vi "dfd_Set MRate Model.vi"(4 "output rounding mode":T5 caption="output round-off mode", 5 "output integer word length":T1, 6 "internal precision":T7, 8 "input iwl":i16=1, 9 "output wl":i16=16, 10 "input wl":i16=16, 11 "multirate filter in":T2={"mMRate_Structure"=enum."CIC", "mMRate_Mode"=0, "mMRate_Factor"=1, "mMRate_FIRParams"={"mMRate_FIR_H"=[], "mMRate_FIR_IsNyquist?"=FALSE, "mMRate_FIR_IsSymmetric?"=FALSE}, "mMRate_CICParams"={"mMRate_CIC_#Stage"=2, "mMRate_CIC_Lag"=1, "mMRate_CIC_Type"=enum."Lowpass"}, "mMRate_Order"=0, "mMRate_Version"="1.0", "mMRate_Comments"="", "mMRate_RationalFactor"={"mMRate_L"=-1, "mMRate_M"=-1}, "mMRate_Fs"=1.0, "mMRate_Quantized?"=FALSE, "mMRate_QFilterGain"=1.0, "mMRate_CoefWl"=16, "mMRate_Scaling"={"mMRate_ScaleByPowerOf2?"=FALSE, "mMRate_ScaleType"=enum."Time Domain 1-Norm"}, "mMRate_InputWl"=0, "mMRate_OutputWl"=0, "mMRate_OutputMode"=enum."Nearest", "mMRate_MultMode"=enum."Truncated", "mMRate_BitPruning"=FALSE, "mMRate_GainWl"=16, "mMRate_OutputFwl"=0, "mMRate_SumIwl"=0, "mMRate_InputIwl "=16, "mMRate_SumWl"=32, "mMRate_CoefIwl"=0} {"mMRate_SumWl" min=1 max=32 step=1; "mMRate_InputIwl" min=1 max=32 step=1; "mMRate_GainWl" min=1 max=32 step=1; "mMRate_OutputWl" min=1 max=32 step=1; "mMRate_InputWl" min=1 max=32 step=1; "mMRate_CoefWl" min=1 max=32 step=1; "mMRate_Mode" items=["Default"=-1, "No Rate Change"=0, "Interpolation"=1, "Decimation"=2, "Interpolated"=3, "Rational"=4]}) -> (3 "multirate filter out":T2={"mMRate_Structure"=enum."CIC", "mMRate_Mode"=0, "mMRate_Factor"=1, "mMRate_FIRParams"={"mMRate_FIR_H"=[], "mMRate_FIR_IsNyquist?"=FALSE, "mMRate_FIR_IsSymmetric?"=FALSE}, "mMRate_CICParams"={"mMRate_CIC_#Stage"=2, "mMRate_CIC_Lag"=1, "mMRate_CIC_Type"=enum."Lowpass"}, "mMRate_Order"=0, "mMRate_Version"="1.0", "mMRate_Comments"="", "mMRate_RationalFactor"={"mMRate_L"=-1, "mMRate_M"=-1}, "mMRate_Fs"=1.0, "mMRate_Quantized?"=FALSE, "mMRate_QFilterGain"=1.0, "mMRate_CoefWl"=16, "mMRate_Scaling"={"mMRate_ScaleByPowerOf2?"=FALSE, "mMRate_ScaleType"=enum."Time Domain 1-Norm"}, "mMRate_InputWl"=0, "mMRate_OutputWl"=0, "mMRate_OutputMode"=enum."Nearest", "mMRate_MultMode"=enum."Truncated", "mMRate_BitPruning"=FALSE, "mMRate_GainWl"=16, "mMRate_OutputFwl"=0, "mMRate_SumIwl"=0, "mMRate_InputIwl "=16, "mMRate_SumWl"=32, "mMRate_CoefIwl"=0} {"mMRate_SumWl" min=1 max=32 step=1; "mMRate_InputIwl" min=1 max=32 step=1; "mMRate_GainWl" min=1 max=32 step=1; "mMRate_OutputWl" min=1 max=32 step=1; "mMRate_InputWl" min=1 max=32 step=1; "mMRate_CoefWl" min=1 max=32 step=1; "mMRate_Mode" items=["Default"=-1, "No Rate Change"=0, "Interpolation"=1, "Decimation"=2, "Interpolated"=3, "Rational"=4]})   [LabVIEW 2017, in "NI_DigFilter_FXP.lvlib"]
uses:
  <vilib>/addons/Digital Filter Design/NI_DigFilter_FXP.lvlib
  <vilib>/addons/Digital Filter Design/_Objects.llb/DFD FXP MRate Internal Precision Mode.ctl
  <vilib>/addons/Digital Filter Design/_Objects.llb/DFD Round-off Mode.ctl
  <vilib>/addons/Digital Filter Design/_Objects.llb/DFD Multirate Filter Obj.ctl
  <vilib>/addons/Digital Filter Design/_Objects.llb/DFD Multirate Mode.ctl
  <vilib>/addons/Digital Filter Design/_Objects.llb/DFD Coef Norm Type.ctl
  <vilib>/addons/Digital Filter Design/_Objects.llb/DFD FXP MRate Multiply Mode.ctl
  <vilib>/addons/Digital Filter Design/_Objects.llb/DFD Output Iwl Obj.ctl
  <vilib>/addons/Digital Filter Design/NI_DigFilterLicensed.lvlib
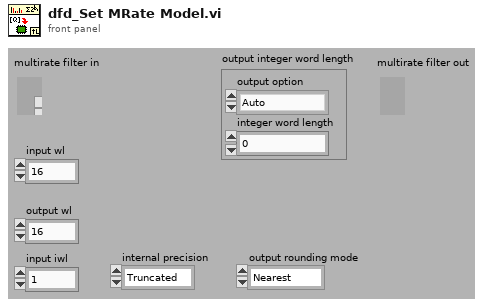
[diagram p1: front panel]
types:
  T1 = typedef "NI_DigFilterLicensed.lvlib/DFD Output Iwl Obj.ctl" = cluster{"output option":enum16{"Auto", "Same As Input", "User Defined"}, "integer word length":i16}
  T2 = typedef "NI_DigFilterLicensed.lvlib/DFD Multirate Filter Obj.ctl" = cluster{"mMRate_Structure":enum16{"CIC", "FIR", "IIR", "Lattice"}, "mMRate_Mode":T3, "mMRate_Factor":i32, "mMRate_FIRParams":cluster{"mMRate_FIR_H":dbl[], "mMRate_FIR_IsNyquist?":bool, "mMRate_FIR_IsSymmetric?":bool}, "mMRate_CICParams":cluster{"mMRate_CIC_#Stage":i32, "mMRate_CIC_Lag":i32, "mMRate_CIC_Type":enum16{"Lowpass", "Highpass"}}, "mMRate_Order":i32, "mMRate_Version":string, "mMRate_Comments":string, "mMRate_RationalFactor":cluster{"mMRate_L":i32, "mMRate_M":i32}, "mMRate_Fs":dbl, "mMRate_Quantized?":bool, "mMRate_QFilterGain":dbl, "mMRate_CoefWl":i16, "mMRate_Scaling":cluster{"mMRate_ScaleByPowerOf2?":bool, "mMRate_ScaleType":T4}, "mMRate_InputWl":i16, "mMRate_OutputWl":i16, "mMRate_OutputMode":T5, "mMRate_MultMode":T6, "mMRate_BitPruning":bool, "mMRate_GainWl":i16, "mMRate_OutputFwl":i16, "mMRate_SumIwl":i16, "mMRate_InputIwl ":i16, "mMRate_SumWl":i16, "mMRate_CoefIwl":i16}
  T3 = typedef "NI_DigFilterLicensed.lvlib/DFD Multirate Mode.ctl" = i16
  T4 = typedef "NI_DigFilterLicensed.lvlib/DFD Coef Norm Type.ctl" = enum16{"No Norm", "Time Domain 1-Norm", "Time Domain 2-Norm", "Time Domain Inf-Norm"}
  T5 = typedef "NI_DigFilterLicensed.lvlib/DFD Round-off Mode.ctl" = enum16{"Nearest", "Truncation"}
  T6 = typedef "NI_DigFilterLicensed.lvlib/DFD FXP MRate Multiply Mode.ctl" = enum16{"Truncated", "Full"}
  T7 = typedef "NI_DigFilterLicensed.lvlib/DFD FXP MRate Internal Precision Mode.ctl" = enum16{"Truncated", "Full"}
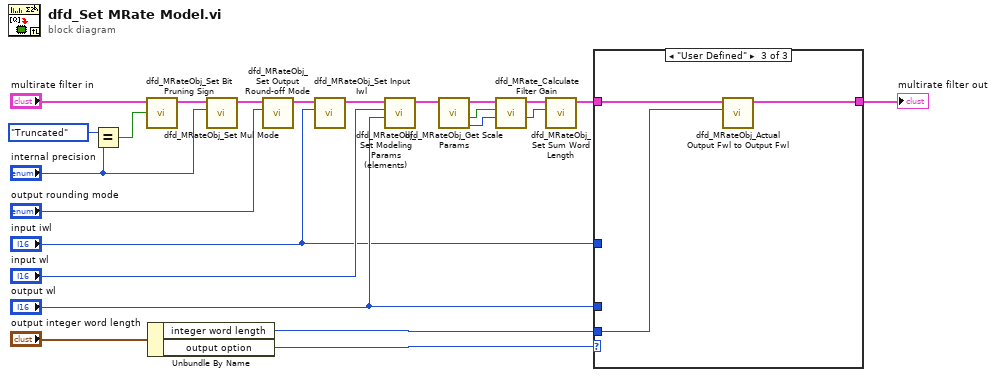
[diagram p0: block diagram]
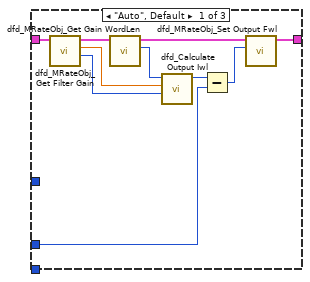
[diagram p2: hidden frame]
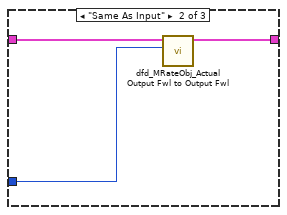
[diagram p3: hidden frame]
diagram:
  n1 = Equal?(x=DFD_FXP_MRate_Internal_Precision_Mode."Truncated", y="internal precision") -> (x = y?=w20:bool)
  n2 = call <vilib>:"dfd_MRateObj_Set Bit Pruning Sign.vi"("bit pruning?"=w20, "multirate filter in"="multirate filter in") -> ("multirate filter out"=w22:T2)  [unwired: 9 out]
  n3 = Unbundle By Name("output integer word length") -> ("integer word length"=w1:i16, "output option"=w2:enum16{"Auto", "Same As Input", "User Defined"})
  n4 = call <vilib>:"dfd_MRateObj_Set Mul Mode.vi"("multiply mode"="internal precision", "multirate filter in"=w22) -> ("multirate filter out"=w23:T2)  [unwired: 9 out]
  n5 = call <vilib>:"dfd_MRateObj_Set Output Round-off Mode.vi"("output round-off mode"="output rounding mode", "multirate filter in"=w23) -> ("multirate filter out"=w7:T2)  [unwired: 9 out]
  n6 = call <vilib>:"dfd_MRateObj_Set Input Iwl.vi"("InputIwl"="input iwl", "multirate filter in"=w7) -> ("multirate filter out"=w6:T2)  [unwired: 9 out]
  n7 = call <vilib>:"dfd_MRateObj_Set Modeling Params (elements).vi"("output wl"="output wl", "input wl"="input wl", "multirate filter in"=w6) -> ("multirate filter out"=w8:T2)  [unwired: 2 in, 6 out]
  n8 = call <vilib>:"dfd_MRateObj_Get Scale Params.vi"("multirate filter in"=w8) -> ("scale type"=w11:T4, "scale by Power of 2?"=w12:bool, "dup multirate filter"=w13:T2)  [unwired: 8 out]
  n9 = call <vilib>:"dfd_MRate_Calculate Filter Gain.vi"("scale type"=w11, "scale by Power of 2?"=w12, "multirate filter in"=w13) -> ("sum iwl"=w10:i16, "dup multirate filter"=w9:T2)  [unwired: 7 out]
  n10 = call <vilib>:"dfd_MRateObj_Set Sum Word Length.vi"("SumIwl"=w10, "multirate filter in"=w9) -> ("multirate filter out"=w14:T2)  [unwired: 1 in, 8 out]
  n11 = case shown="\"User Defined\"" w2 {
    tunnel: [w29 w35 w38] -> w17
    tunnel: w14 -> [w25 w36 w39]
    tunnel: "output wl" -> [w24 _ _]
    tunnel: "input iwl" -> [_ w34 _]
    tunnel: w1 -> [_ _ w37]
    frame "Auto", Default {
      n12 = call <vilib>:"dfd_MRateObj_Get Filter Gain.vi"("multirate filter in"=w25) -> ("sum iwl"=w31:i16, "gain"=w32:dbl, "dup multirate filter"=w33:T2)  [unwired: 8 out]
      n13 = call <vilib>:"dfd_MRateObj_Get Gain WordLen.vi"("multirate filter in"=w33) -> ("gain wl"=w27:i16, "dup multirate filter"=w26:T2)  [unwired: 9 out]
      n14 = call <vilib>:"dfd_Calculate Output Iwl.vi"("sum iwl"=w31, "gain value"=w32, "gain wl"=w27) -> ("output iwl"=w30:i16)  [unwired: 8 out]
      n15 = Subtract(x=w30, y=w24) -> (x-y=w28:i16)
      n16 = call <vilib>:"dfd_MRateObj_Set Output Fwl.vi"("output fwl"=w28, "multirate filter in"=w26) -> ("multirate filter out"=w29:T2)  [unwired: 9 out]
    }
    frame "Same As Input" {
      n17 = call <vilib>:"dfd_MRateObj_Actual Output Fwl to Output Fwl.vi"("actual output iwl"=w34, "multirate filter in"=w36) -> ("multirate filter out"=w35:T2)  [unwired: 9 out]
    }
    frame "User Defined" {
      n18 = call <vilib>:"dfd_MRateObj_Actual Output Fwl to Output Fwl.vi"("actual output iwl"=w37, "multirate filter in"=w39) -> ("multirate filter out"=w38:T2)  [unwired: 9 out]
    }
  }
  "multirate filter out" <- w17
